vi "CP_meas_freq.vi"() -> ()   [LabVIEW 2014]
uses:
  <vilib>/Utility/file.llb/Write To Spreadsheet File (DBL).vi
  <vilib>/Utility/file.llb/Read From Spreadsheet File (DBL).vi
  <vilib>/gmath/NumericalOptimization/Nonlinear Curve Fit LM formula string.vi
  <vilib>/Analysis/NI_AALBase.lvlib
  <vilib>/gmath/NI_Gmath.lvlib
panel:
  in  "semester":string(combo)="ws17"
  out "error A":dbl format="%.1f"
  out "error T2":dbl format="%.1f"
  out "fit A":dbl format="%.1f"
  out "fit T2[ms]":dbl format="%.1f"
  out "?":dbl[](array[numeric])=[50.0, 20.0] format="%.1f"
  out "XY Graph":cluster{"Y":dbl[], "Y":dbl[]}[](graph)
  out "error":dbl[](array[numeric])=[0.0562386778791667, 0.05751523427745943, 0.055593914838308334, 0.05045808967893851, 0.060948992666645566] format="%.2g"
  out "mean":dbl[](array[numeric])=[1.326611951410732, 0.9785955332997016, 0.994717486473613, 0.8943892146676372, 0.898716105209141] format="%.2g"
  out "meas done":i32=10
  out "Amplitude":cluster{"Y":dbl[], "Y":dbl[]}[](graph)
  in  "SE time":u32[](array[numeric])=[120, 200, 280, 360, 440]
  in  "nr of SE":u32
  out "hlim":dbl=1195.121951219512 format="%#.1f"
  out "llim":dbl=848.780487804878 format="%#.1f"
  out "spin echo\nsignal":dbl
  in  "time-out":u32=6
  in  "gain":u32=1000
  out "Fourier\nspectrum":cluster{"Y":dbl[], "Y":dbl[]}[](graph)
  in  "del T (+-)":u32=10
  in  "folder":string
  in  "fit:":bool=TRUE
  in  "many measurements:":bool=TRUE
  in  "data file":string
  out "zoom":cluster{"Y":dbl[], "Y":dbl[]}[](graph)
  in  "scan freq [kHz]":u32=10
  in  "meas. time":u32=800
  in  "number meas":i32=10
  in  "spin echo time":u32=120
  in  "single measurement:":bool=TRUE
  in  "stop":bool=TRUE
  # "1)"
  # "2)"
  # "3)"
  # "init values"
  # "T2_i[ms]"
  # "A_i"
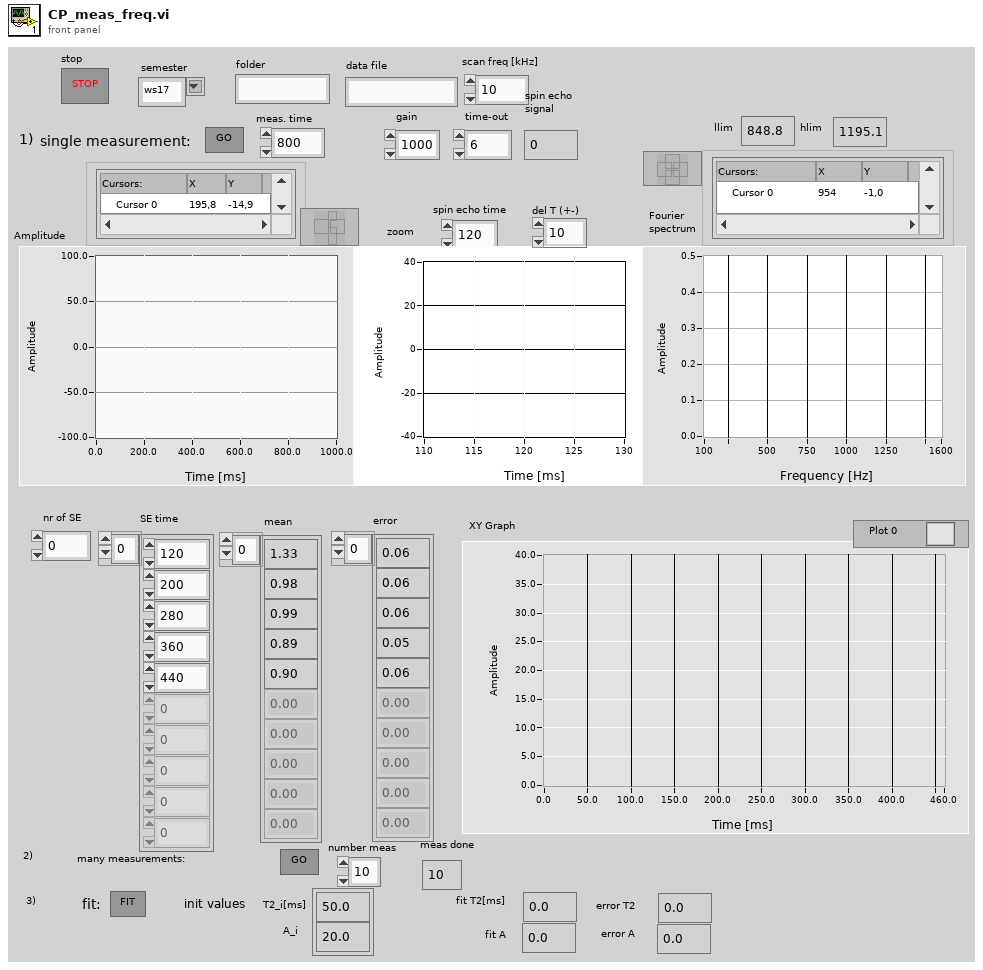
[diagram p1: front panel]
types:
  T1 = cluster{"model":string, "Parameters":string[], "x":string}
  T2 = typedef "LVCursorListTypeDef.ctl" = cluster{"Name":string, "Color":u32, "Style":u8, "Point Style":u8, "Name Visible":bool, "Allow Drag":bool, "Cursor Mode":u32, "Plot":i32, "Index":i32, "Position":cluster{"X":dbl, "Y":dbl}, "X Scale":u32, "Y Scale":u32, "Watch Plots":i32[], "Watch All Plots":bool, "Plot Area":i32, "Label Offset":cluster{"X":dbl, "Y":dbl}}[]
  T3 = typedef "NI_Matrix.lvlib/RealMatrix.ctl" = dbl[][]
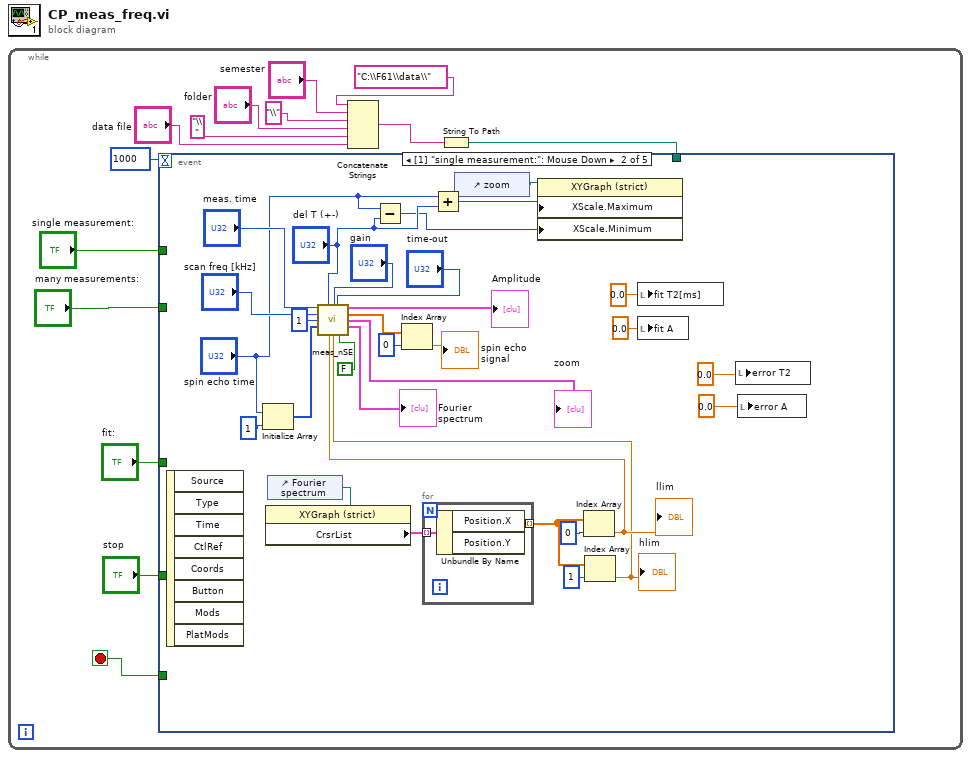
[diagram p0: block diagram]
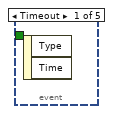
[diagram p2: hidden frame]
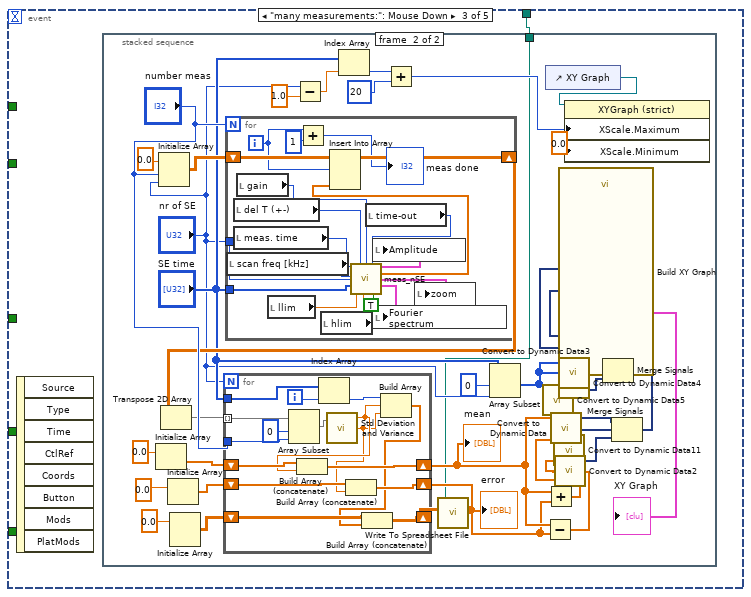
[diagram p3: hidden frame]
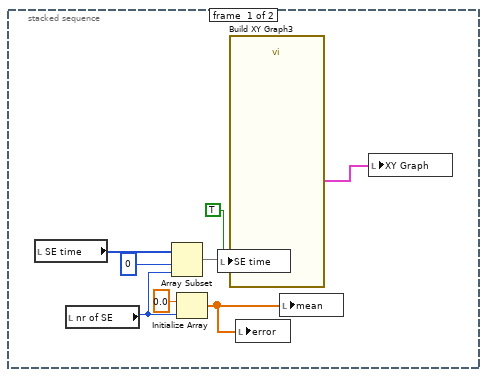
[diagram p4: hidden frame]
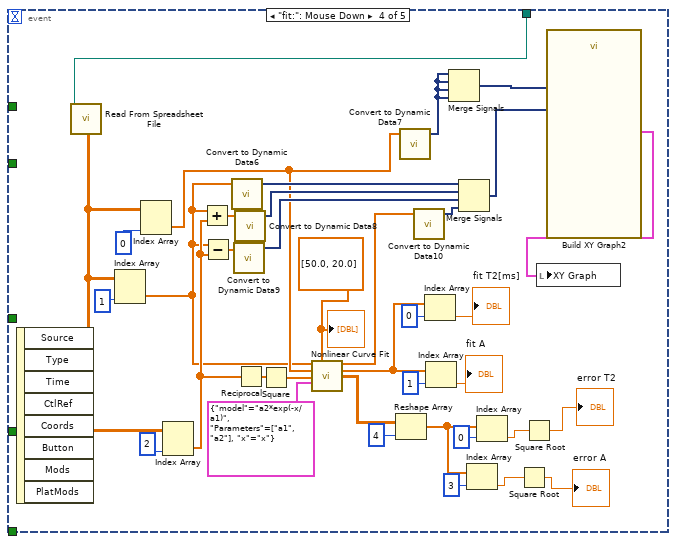
[diagram p5: hidden frame]
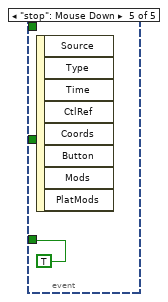
[diagram p6: hidden frame]
diagram:
  n1 = while {
    stop <- w8 stop-if-true
    n2 = Concatenate Strings("C:\\F61\\data\\", "semester", "\\" ("string"), "folder", "\\" ("string"), "data file") -> (w13:string)
    n3 = String To Path(string=w13) -> (path=w12:path)
    n4 = event shown="[1] \"single measurement:\": Mouse Down" {
      selector: _ -> [_ _ _ _ _]
      dyn-events: _ -> [_ _ _ _ _]
      timeout: 1000 -> [_ _ _ _ _]
      tunnel: "single measurement:" -> [_ _ _ _ _]
      tunnel: w12 -> [_ _ w47 w147 _]
      tunnel: "many measurements:" -> [_ _ _ _ _]
      tunnel: "fit:" -> [_ _ _ _ _]
      tunnel: "stop" -> [_ _ _ _ _]
      tunnel: [_ _ _ _ TRUE ("stop")] -> w8
      event Timeout {
        n5 = event-data() -> ()  [unwired: 1 in, 2 out]
      }
      event "single measurement:": Mouse Down {
        n6 = event-data() -> ()  [unwired: 1 in, 8 out]
        n7 = Initialize Array("spin echo time", 1 ("dimension size")) -> (w34:u32[])
        n8 = control-ref of="Fourier\nspectrum"() -> (w44:refnum<vi>)
        n9 = property class="XYGraph (strict)"(reference=w44) -> ("CrsrList"=w43:T2)  [unwired: 1 in, 2 out]
        n10 = Subtract(x="spin echo time", y="del T (+-)") -> (x-y=w19:u32)
        n11 = for {
          tunnel: w43 -> [w46] mode=indexing
          tunnel: [w45] -> w42 mode=indexing
          n12 = Unbundle By Name(w46) -> ("Position.X"=w45:dbl)  [unwired: 1 out]
        }
        n13 = Add(x="spin echo time", y="del T (+-)") -> (x+y=w20:u32)
        n14 = control-ref of="zoom"() -> (w39:refnum<vi>)
        n15 = property class="XYGraph (strict)"(reference=w39, "XScale.Maximum"=w20, "XScale.Minimum"=w19) -> ()  [unwired: 1 in, 2 out]
        n16 = Index Array(array=w42, index=0) -> (element=w33:dbl)
        "llim" <- w33
        n17 = Index Array(array=w42, index=1) -> (element=w32:dbl)
        "hlim" <- w32
        n18 = call "meas_nSE.vi"("meas. time [ms]"="meas. time", "del T (+-) ][ms]"="del T (+-)", "gainfac"="gain", "time out [s]"="time-out", "scan freq [kHz]"="scan freq [kHz]", "nr of SE"=u32 1, "SE-times"=w34, "llim"=w33, "hlim"=w32, "Do-nSE"=FALSE) -> ("Amplitude"=→"Amplitude":cluster{"Y":dbl[], "Y":dbl[]}[], "SE-arr"=w25:dbl[], "zoom window on spin echo nr:"=→"zoom":cluster{"Y":dbl[], "Y":dbl[]}[], "Spin echo (freq)"=→"Fourier\nspectrum":cluster{"Y":dbl[], "Y":dbl[]}[])  [unwired: 2 out]
        n19 = Index Array(array=w25, index=0) -> (element=→"spin echo\nsignal":dbl)
        n20 = local write "fit T2[ms]"(0.0 ("fit T2[ms]")) -> ()
        n21 = local write "fit A"(0.0 ("fit A")) -> ()
        n22 = local write "error T2"(0.0 ("error T2")) -> ()
        n23 = local write "error A"(0.0 ("error A")) -> ()
      }
      event "many measurements:": Mouse Down {
        n24 = event-data() -> ()  [unwired: 1 in, 8 out]
        n25 = stacked-sequence {
          tunnel: w47 -> [_ w57]
          frame #0 {
            n26 = local read "SE time"() -> (w51:u32[])
            n27 = local read "nr of SE"() -> (w49:u32)
            n28 = Array Subset(array=w51, index=0, length=w49) -> (w48:u32[])
            n29 = Initialize Array(0.0 ("element"), w49) -> (w52:dbl[])
            n30 = local write "SE time"(w48) -> ()
            n31 = call "Build XY Graph3"("Reset"=TRUE) -> ("XY Graph"=w55:cluster{"X":dbl[], "Y":dbl[]}[])  [unwired: 9 in, 1 out]
            n32 = local write "error"(w52) -> ()
            n33 = local write "mean"(w52) -> ()
            n34 = local write "XY Graph"(w55) -> ()
          }
          frame #1 {
            n35 = Initialize Array(0.0 ("element")) -> (w87:dbl[])  [unwired: 1 in]
            n36 = Initialize Array(0.0 ("element"), "number meas", "nr of SE") -> (w91:dbl[][])
            n37 = Initialize Array(0.0 ("element")) -> (w86:dbl[])  [unwired: 1 in]
            n38 = Initialize Array(0.0 ("element")) -> (w59:dbl[][])  [unwired: 2 in]
            n39 = for {
              N: "number meas" -> [_]
              shift-right: [w114] -> w88
              shift-left: w91 -> [w115]
              tunnel: "nr of SE" -> [w125]
              tunnel: "SE time" -> [w124]
              i -> [w111]
              n40 = local read "scan freq [kHz]"() -> (w126:u32)
              n41 = local read "del T (+-)"() -> (w120:u32)
              n42 = local read "meas. time"() -> (w127:u32)
              n43 = local read "gain"() -> (w112:u32)
              n44 = local read "llim"() -> (w123:dbl)
              n45 = Add(x=w111, y=1) -> (x+y=→"meas done":i32)
              n46 = local read "hlim"() -> (w122:dbl)
              n47 = local read "time-out"() -> (w119:u32)
              n48 = call "meas_nSE.vi"("meas. time [ms]"=w127, "del T (+-) ][ms]"=w120, "gainfac"=w112, "time out [s]"=w119, "scan freq [kHz]"=w126, "nr of SE"=w125, "SE-times"=w124, "llim"=w123, "hlim"=w122, "Do-nSE"=TRUE) -> ("Amplitude"=w116:cluster{"Y":dbl[], "Y":dbl[]}[], "SE-arr"=w113:dbl[], "zoom window on spin echo nr:"=w118:cluster{"Y":dbl[], "Y":dbl[]}[], "Spin echo (freq)"=w117:cluster{"Y":dbl[], "Y":dbl[]}[])  [unwired: 2 out]
              n49 = Insert Into Array(array=w115, index (row)=w111, new element=w113) -> (w114:dbl[][])  [unwired: 1 in]
              n50 = local write "Amplitude"(w116) -> ()
              n51 = local write "Fourier\nspectrum"(w117) -> ()
              n52 = local write "zoom"(w118) -> ()
            }
            n53 = Transpose 2D Array(2D array=w88) -> (transposed array=w89:dbl[][])
            n54 = for {
              N: "nr of SE" -> [_]
              tunnel: w89 -> [w108] mode=indexing
              tunnel: "number meas" -> [w107]
              shift-right: [w103] -> w75
              shift-left: w87 -> [w104]
              shift-right: [w101] -> w74
              shift-left: w86 -> [w102]
              tunnel: "SE time" -> [w100]
              shift-right: [w94] -> w56
              shift-left: w59 -> [w95]
              i -> [w99]
              n55 = Array Subset(array=w108, index=0, length=w107) -> (w105:dbl[])
              n56 = Index Array(array=w100, index=w99) -> (element=w96:u32)
              n57 = call <vilib>:"Std Deviation and Variance.vi"("X"=w105) -> ("mean"=w98:dbl, "standard deviation"=w97:dbl)  [unwired: 1 in, 1 out]
              n58 = Build Array (concatenate)(w104, w98) -> (w103:dbl[])
              n59 = Build Array (concatenate)(w102, w97) -> (w101:dbl[])
              n60 = Build Array(w96, w98, w97) -> (w93:dbl[])
              n61 = Build Array (concatenate)(w95, w93) -> (w94:dbl[][])
            }
            "mean" <- w75
            "error" <- w74
            n62 = Subtract(x="nr of SE", y=1.0) -> (x-y=w64:dbl)
            n63 = Index Array(array="SE time", index=w64) -> (element=w63:u32)
            n64 = Add(x=w63, y=u32 20) -> (x+y=w61:u32)
            n65 = call-poly <vilib>:"Write To Spreadsheet File.vi"("2D data"=w56, "file path (dialog if empty)"=w57) -> ()  [unwired: 6 in, 1 out]
            n66 = Array Subset(array="SE time", index=0 ("length"), length="nr of SE") -> (w79:u32[])
            n67 = call "Convert to Dynamic Data5"("Array"=w79) -> ("Dynamic Data Type"=w78:dynamicdata)  [unwired: 3 in]
            n68 = Subtract(x=w75, y=w74) -> (x-y=w72:dbl[])
            n69 = control-ref of="XY Graph"() -> (w67:refnum<vi>)
            n70 = Add(x=w75, y=w74) -> (x+y=w73:dbl[])
            n71 = call "Convert to Dynamic Data"("Array"=w75) -> ("Dynamic Data Type"=w77:dynamicdata)  [unwired: 3 in]
            n72 = call "Convert to Dynamic Data11"("Array"=w73) -> ("Dynamic Data Type"=w76:dynamicdata)  [unwired: 3 in]
            n73 = call "Convert to Dynamic Data2"("Array"=w72) -> ("Dynamic Data Type"=w82:dynamicdata)  [unwired: 3 in]
            n74 = call "Convert to Dynamic Data3"("Array"=w79) -> ("Dynamic Data Type"=w81:dynamicdata)  [unwired: 3 in]
            n75 = call "Convert to Dynamic Data4"("Array"=w79) -> ("Dynamic Data Type"=w80:dynamicdata)  [unwired: 3 in]
            n76 = property class="XYGraph (strict)"(reference=w67, "XScale.Maximum"=w61, "XScale.Minimum"=0.0 ("X Scale.Range:Minimum")) -> ()  [unwired: 1 in, 2 out]
            n77 = Merge Signals(w81, w80, w78) -> (w70:dynamicdata)
            n78 = Merge Signals(w77, w76, w82) -> (w69:dynamicdata)
            n79 = call "Build XY Graph"("Y Input"=w69, "X Input"=w70) -> ("XY Graph"=→"XY Graph":cluster{"X":dbl[], "Y":dbl[]}[])  [unwired: 8 in, 1 out]
          }
        }
      }
      event "fit:": Mouse Down {
        w143 = dbl[] [50.0, 20.0] ("initial parameters")
        n80 = event-data() -> ()  [unwired: 1 in, 8 out]
        n81 = call-poly <vilib>:"Read From Spreadsheet File.vi"("file path (dialog if empty)"=w147) -> ("all rows"=w164:dbl[][])  [unwired: 6 in, 4 out]
        n82 = Index Array(array=w164, index (col)=1 ("index (row)")) -> (element=w145:dbl[])  [unwired: 1 in]
        n83 = Index Array(array=w164, index (col)=0 ("index (row)")) -> (element=w148:dbl[])  [unwired: 1 in]
        n84 = Index Array(array=w164, index (col)=2 ("index (row)")) -> (element=w153:dbl[])  [unwired: 1 in]
        n85 = Add(x=w145, y=w153) -> (x+y=w157:dbl[])
        n86 = Subtract(x=w145, y=w153) -> (x-y=w156:dbl[])
        n87 = call "Convert to Dynamic Data6"("Array"=w145) -> ("Dynamic Data Type"=w158:dynamicdata)  [unwired: 3 in]
        n88 = call "Convert to Dynamic Data9"("Array"=w156) -> ("Dynamic Data Type"=w154:dynamicdata)  [unwired: 3 in]
        n89 = call "Convert to Dynamic Data8"("Array"=w157) -> ("Dynamic Data Type"=w155:dynamicdata)  [unwired: 3 in]
        n90 = Reciprocal(x=w153) -> (1/x=w152:dbl[])
        n91 = Square(x=w152) -> (x^2=w151:dbl[])
        n92 = call-poly <vilib>:"Nonlinear Curve Fit.vi"("Y"=w145, "initial parameters"=w143, "X"=w148, "Weight"=w151, "model description"=T1 {"model"="a2*exp(-x/a1)", "Parameters"=["a1", "a2"], "x"="x"}) -> ("best nonlinear fit"=w150:dbl[], "best fit parameters"=w141:dbl[], "covariance"=w137:T3)  [unwired: 6 in, 2 out]
        n93 = Reshape Array(w137, 4 ("dimension size")) -> (w135:dbl[])
        n94 = call "Convert to Dynamic Data7"("Array"=w148) -> ("Dynamic Data Type"=w146:dynamicdata)  [unwired: 3 in]
        n95 = call "Convert to Dynamic Data10"("Array"=w150) -> ("Dynamic Data Type"=w149:dynamicdata)  [unwired: 3 in]
        n96 = Index Array(array=w141, index=0) -> (element=→"fit T2[ms]":dbl)
        n97 = Index Array(array=w141, index=1) -> (element=→"fit A":dbl)
        n98 = Merge Signals(w146, w146, w146, w146) -> (w160:dynamicdata)
        n99 = Merge Signals(w158, w155, w154, w149) -> (w159:dynamicdata)
        n100 = Index Array(array=w135, index=3) -> (element=w130:dbl)
        n101 = Index Array(array=w135, index=0) -> (element=w132:dbl)
        n102 = Square Root(x=w130) -> (sqrt(x)=→"error A":dbl)
        n103 = Square Root(x=w132) -> (sqrt(x)=→"error T2":dbl)
        n104 = call "Build XY Graph2"("Y Input"=w159, "X Input"=w160) -> ("XY Graph"=w128:cluster{"Y":dbl[], "Y":dbl[]}[])  [unwired: 8 in, 1 out]
        n105 = local write "XY Graph"(w128) -> ()
        "?" <- w143
      }
      event "stop": Mouse Down {
        n106 = event-data() -> ()  [unwired: 1 in, 8 out]
      }
    }
  }
